vi "DSF.Engine.Interface.Plugin.Read.Command.vi"(8 "error in (no error)":errorcluster, 9 "timeout in ms (0)":i32, 11 "Plugin Interface in":refnum<class "DSF.Engine.Interface.Plugin.lvclass">) -> (0 "error out":errorcluster, 1 "empty?":bool, 2 "command":T1, 3 "Plugin Interface out":refnum<class "DSF.Engine.Interface.Plugin.lvclass">, 4 "# elements":u32)   [LabVIEW 2016, in "DSF.Engine.lvlib" / "DSF.Engine.Interface.Plugin.lvclass"]
uses:
  DSF.Engine.Interface.Plugin.lvclass
  C:/Git/Sourcetree/DSF/Source/Engine/Classes/Interface/DSF.Engine.Interface.lvclass
  DSF.Engine.Interface.Plugin.Command Data.ctl
  DSF.Engine.Interface.Plugin.Command.ctl
  DSF.Engine.Interface.lvclass/DSF.Engine.Interface.ctl
  DSF.Engine.Interface.lvclass
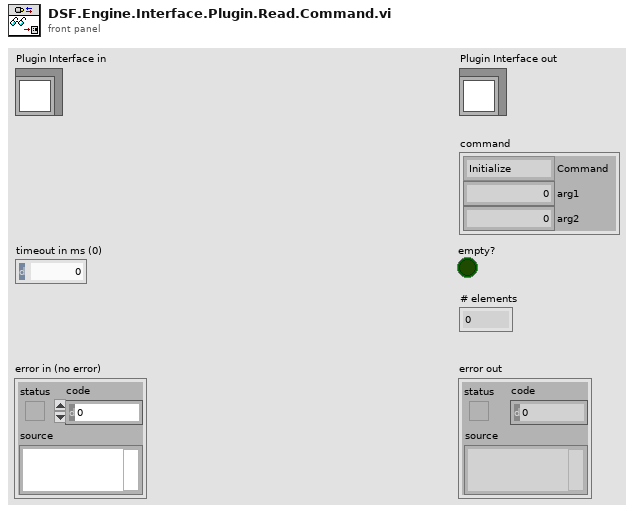
[diagram p1: front panel]
types:
  T1 = typedef "DSF.Engine.lvlib/DSF.Engine.Interface.Plugin.lvclass/DSF.Engine.Interface.Plugin.Command Data.ctl" = cluster{"Command":T2, "arg1":u64, "arg2":u64}
  T2 = typedef "DSF.Engine.lvlib/DSF.Engine.Interface.Plugin.lvclass/DSF.Engine.Interface.Plugin.Command.ctl" = enum8{"Initialize", "Process Rx", "Process Tx", "Shutdown"}
  T3 = typedef "DSF.Engine.lvlib/DSF.Engine.Interface.lvclass/DSF.Engine.Interface.RT FIFO.Ref.16B.ctl" = refnum<k33>
  T4 = typedef "DSF.Engine.lvlib/DSF.Engine.Interface.lvclass/DSF.Engine.Interface.RT FIFO.Data.16B.ctl" = cluster{"Command":u8, "Payload":T5}
  T5 = typedef "DSF.Engine.lvlib/DSF.Engine.Interface.lvclass/DSF.Engine.Interface.RT FIFO.Payload.16B.ctl" = cluster{"arg1":u64, "arg2":u64}
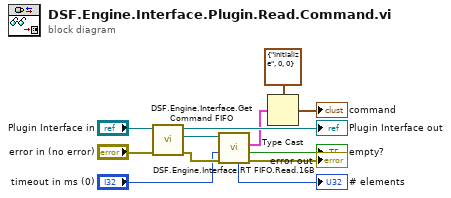
[diagram p0: block diagram]
diagram:
  n1 = call "DSF.Engine.Interface.Get Command FIFO.vi"("error in (no error)"="error in (no error)", "Interface in"="Plugin Interface in") -> ("error out"=w9:errorcluster, "Command FIFO"=w10:T3, "Interface out"=→"Plugin Interface out":refnum<class "DSF.Engine.Interface.Plugin.lvclass">)  [unwired: 7 in]
  n2 = call "DSF.Engine.Interface.RT FIFO.Read.16B.vi"("error in (no error)"=w9, "timeout in ms (0)"="timeout in ms (0)", "RT FIFO in"=w10) -> ("error out"=→"error out":errorcluster, "empty?"=→"empty?":bool, "element out"=w3:T4, "# elements"=→"# elements":u32)  [unwired: 4 in, 1 out]
  n3 = Type Cast(type=T1 {"Command"=enum."Initialize", "arg1"=0, "arg2"=0} ("Plugin Command"), x=w3) -> (*(type *) &x=→"command":T1)
